vi "Set Table Background Color.vi"(8 "Error In":errorcluster caption="错误输入", 10 "活动单元格":cluster{"活动单元格:活动单元格":T1, "活动单元格:单元格背景色":u32}[](array[cluster]), 11 "Tbl引用句柄":refnum<vi>) -> (0 "Error Out":errorcluster caption="错误输出")   [LabVIEW 2015, in "Utility VIs.lvlib"]
uses:
  Utility VIs.lvlib
  <vilib>/Utility/miscctls.llb/LVRowAndColumnTypeDef.ctl
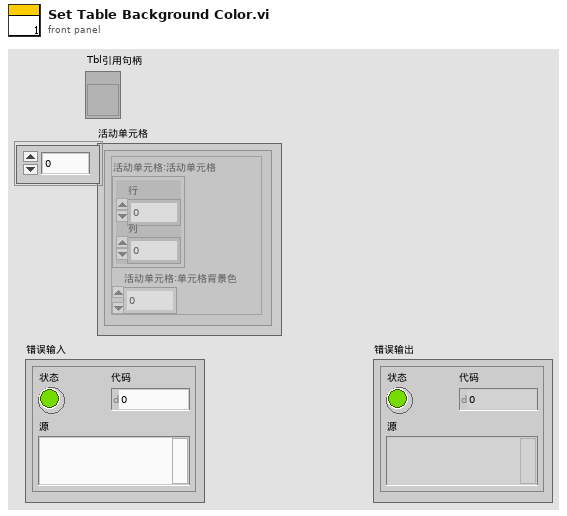
[diagram p1: front panel]
types:
  T1 = typedef "LVRowAndColumnTypeDef.ctl" = cluster{"Row":i32, "Column":i32}
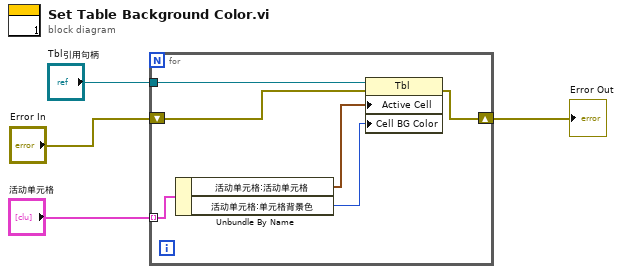
[diagram p0: block diagram]
diagram:
  n1 = for {
    tunnel: "Tbl引用句柄" -> [w10]
    tunnel: "活动单元格" -> [w9] mode=indexing
    shift-right: [w6] -> w1
    shift-left: "Error In" -> [w5]
    n2 = Unbundle By Name(w9) -> ("活动单元格:活动单元格"=w8:T1, "活动单元格:单元格背景色"=w7:u32)
    n3 = property class="Tbl"(reference=w10, error in=w5, "Active Cell"=w8, "Cell BG Color"=w7) -> (error out=w6:errorcluster)  [unwired: 1 out]
  }
  "Error Out" <- w1
